vi "Rise_Fall_Time.vi"(0 "Analog_Waveform":waveform(dbl)(graph)={"t0"=timestamp(0 s since 1904-01-01), "dt"=1e-06, "Y"=array[5000 elements]}, 5 "Amplitude(V)":dbl=5.0) -> (4 "Rise_Time (s)":dbl, 6 "Fall_Time (s)":dbl)   [LabVIEW 2023]
uses:
  Controls/Indexes_Min_Max_Points.ctl
  Controls/Index_Select.ctl
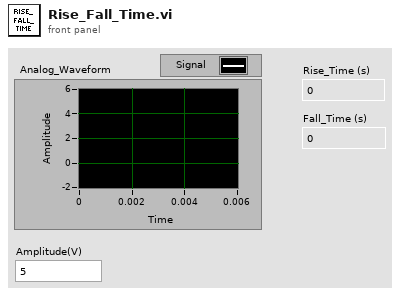
[diagram p1: front panel]
types:
  T1 = typedef "Index_Select.ctl" = enum16{"Wait_for_0", "Index_RTS", "Index_RTE", "Index_FTS", "Index_FTE"}
  T2 = typedef "Indexes_Min_Max_Points.ctl" = cluster{"Index_RTS":i32, "Index_RTE":i32, "Index_FTS":i32, "Index_FTE":i32}
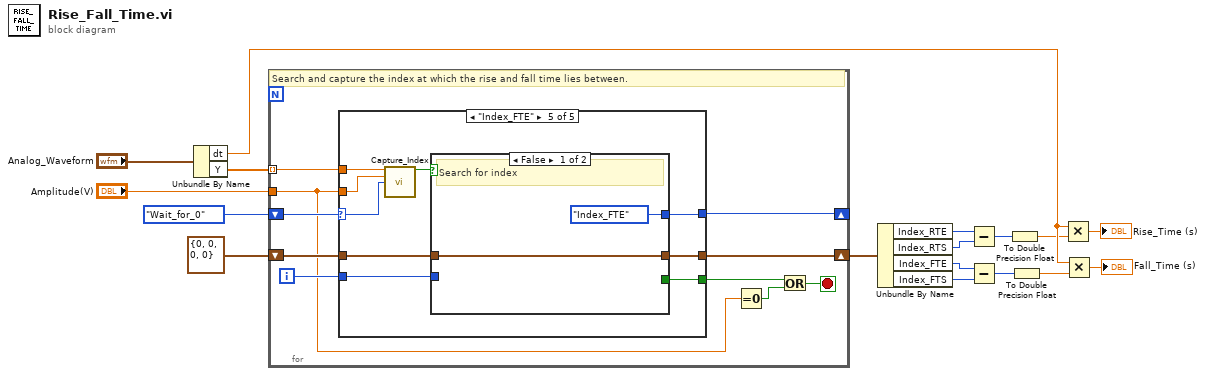
[diagram p0: block diagram]
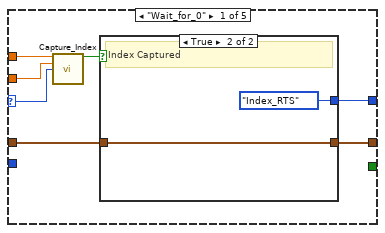
[diagram p2: hidden frame]
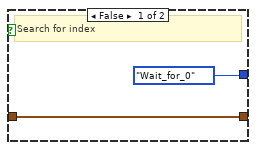
[diagram p3: hidden frame]
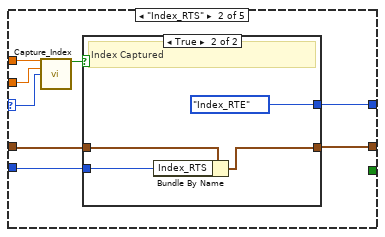
[diagram p4: hidden frame]
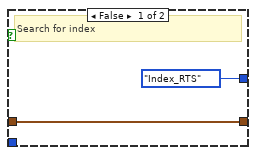
[diagram p5: hidden frame]
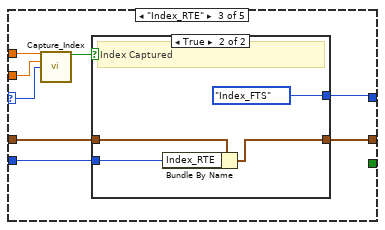
[diagram p6: hidden frame]
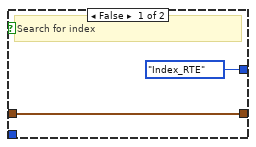
[diagram p7: hidden frame]
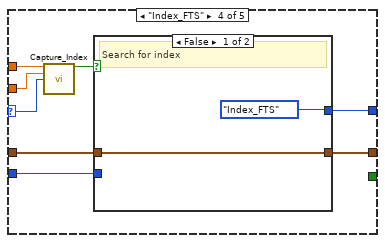
[diagram p8: hidden frame]
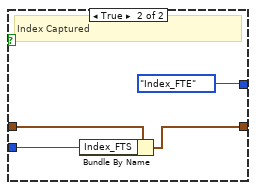
[diagram p9: hidden frame]
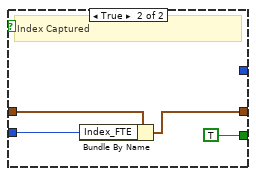
[diagram p10: hidden frame]
diagram:
  n1 = Unbundle By Name("Analog_Waveform") -> ("dt"=w6:dbl, "Y"=w16:dbl[])
  n2 = for {
    tunnel: w16 -> [w25] mode=indexing
    tunnel: "Amplitude(V)" -> [w18]
    shift-right: [w26] -> w12
    shift-left: T2 {"Index_RTS"=0, "Index_RTE"=0, "Index_FTS"=0, "Index_FTE"=0} -> [w27]
    shift-right: [w22] -> _
    shift-left: Index_Select."Wait_for_0" -> [w23]
    i -> [w24]
    stop <- w20 stop-if-true
    # "Search and capture the index at which the rise and fall time lies between."
    n3 = case shown="\"Index_FTE\"" w23 {
      selector: w23 -> [w29 w40 w54 w68 w82]
      tunnel: w27 -> [w32 w46 w60 w74 w89]
      tunnel: [w33 w43 w59 w71 w86] -> w26
      tunnel: w25 -> [w31 w42 w56 w70 w84]
      tunnel: w18 -> [w30 w41 w55 w69 w83]
      tunnel: w24 -> [_ w45 w58 w73 w88]
      tunnel: [_ _ _ _ w85] -> w21
      tunnel: [w34 w44 w57 w72 w87] -> w22
      frame "Wait_for_0" {
        n4 = call "Capture_Index.vi"("Y"=w31, "Amplitude(V)"=w30, "Index_Select"=w29) -> ("Capture?"=w28:bool)  [unwired: 12 in]
        n5 = case shown="True" w28 {
          tunnel: w32 -> [w36 w38]
          tunnel: [w36 w38] -> w33
          tunnel: [Index_Select."Wait_for_0" Index_Select."Index_RTS"] -> w34
          frame False {
            # "Search for index"
          }
          frame True {
            # "Index Captured"
          }
        }
      }
      frame "Index_RTS" {
        n6 = call "Capture_Index.vi"("Y"=w42, "Amplitude(V)"=w41, "Index_Select"=w40) -> ("Capture?"=w39:bool)  [unwired: 12 in]
        n7 = case shown="True" w39 {
          tunnel: w46 -> [w48 w52]
          tunnel: [w48 w51] -> w43
          tunnel: w45 -> [_ w50]
          tunnel: [Index_Select."Index_RTS" Index_Select."Index_RTE"] -> w44
          frame False {
            # "Search for index"
          }
          frame True {
            # "Index Captured"
            n8 = Bundle By Name(cluster=w52, "Index_RTS"=w50) -> (w51:T2)
          }
        }
      }
      frame "Index_RTE" {
        n9 = call "Capture_Index.vi"("Y"=w56, "Amplitude(V)"=w55, "Index_Select"=w54) -> ("Capture?"=w53:bool)  [unwired: 12 in]
        n10 = case shown="True" w53 {
          tunnel: w60 -> [w62 w66]
          tunnel: [w62 w65] -> w59
          tunnel: w58 -> [_ w64]
          tunnel: [Index_Select."Index_RTE" Index_Select."Index_FTS"] -> w57
          frame False {
            # "Search for index"
          }
          frame True {
            # "Index Captured"
            n11 = Bundle By Name(cluster=w66, "Index_RTE"=w64) -> (w65:T2)
          }
        }
      }
      frame "Index_FTS" {
        n12 = call "Capture_Index.vi"("Y"=w70, "Amplitude(V)"=w69, "Index_Select"=w68) -> ("Capture?"=w67:bool)  [unwired: 12 in]
        n13 = case shown="False" w67 {
          tunnel: w74 -> [w75 w80]
          tunnel: [w75 w79] -> w71
          tunnel: w73 -> [_ w78]
          tunnel: [Index_Select."Index_FTS" Index_Select."Index_FTE"] -> w72
          frame False {
            # "Search for index"
          }
          frame True {
            # "Index Captured"
            n14 = Bundle By Name(cluster=w80, "Index_FTS"=w78) -> (w79:T2)
          }
        }
      }
      frame "Index_FTE" {
        n15 = call "Capture_Index.vi"("Y"=w84, "Amplitude(V)"=w83, "Index_Select"=w82) -> ("Capture?"=w81:bool)  [unwired: 12 in]
        n16 = case shown="False" w81 {
          tunnel: w89 -> [w91 w95]
          tunnel: [w91 w94] -> w86
          tunnel: w88 -> [_ w93]
          tunnel: [Index_Select."Index_FTE" _] -> w87
          tunnel: [_ TRUE] -> w85
          frame False {
            # "Search for index"
          }
          frame True {
            # "Index Captured"
            n17 = Bundle By Name(cluster=w95, "Index_FTE"=w93) -> (w94:T2)
          }
        }
      }
    }
    n18 = Equal To 0?(x=w18) -> (x = 0?=w19:bool)
    n19 = Or(x=w21, y=w19) -> (x .or. y?=w20:bool)
  }
  n20 = Unbundle By Name(w12) -> ("Index_RTE"=w11:i32, "Index_RTS"=w8:i32, "Index_FTE"=w10:i32, "Index_FTS"=w9:i32)
  n21 = Subtract(x=w11, y=w8) -> (x-y=w7:i32)
  n22 = Subtract(x=w10, y=w9) -> (x-y=w5:i32)
  n23 = To Double Precision Float(number=w7) -> (double precision float=w4:dbl)
  n24 = To Double Precision Float(number=w5) -> (double precision float=w3:dbl)
  n25 = Multiply(x=w6, y=w4) -> (x*y=→"Rise_Time (s)":dbl)
  n26 = Multiply(x=w6, y=w3) -> (x*y=→"Fall_Time (s)":dbl)
